vi "Make_Periodic.vi"(1 "Input Array":i64[](array[numeric])=[1, 0], 4 "Periods":u64=1) -> (15 "Output Array":i64[](array[numeric])=[1, 0], 18 "Output Length":u64=2)   [LabVIEW 2014]
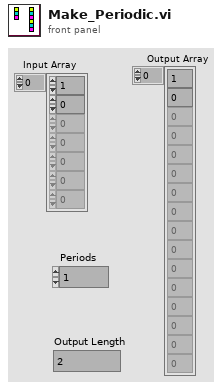
[diagram p1: front panel]
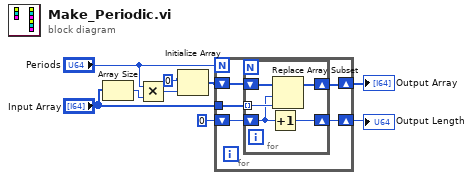
[diagram p0: block diagram]
diagram:
  n1 = Array Size(array="Input Array") -> (size(s)=w6:i32)
  n2 = Multiply(x="Periods", y=w6) -> (x*y=w4:u64)
  n3 = Initialize Array(i64 0 ("element"), w4) -> (w8:i64[])
  n4 = for {
    N: "Periods" -> [_]
    shift-right: [w12] -> w3
    shift-left: w8 -> [w13]
    tunnel: "Input Array" -> [w14]
    shift-right: [w10] -> w1
    shift-left: u64 0 ("element") -> [w11]
    n5 = for {
      tunnel: w14 -> [w17] mode=indexing
      shift-right: [w18] -> w12
      shift-left: w13 -> [w19]
      shift-right: [w16] -> w10
      shift-left: w11 -> [w15]
      n6 = Increment(x=w15) -> (x+1=w16:u64)
      n7 = Replace Array Subset(array=w19, new element=w17, index=w15) -> (w18:i64[])
    }
  }
  "Output Array" <- w3
  "Output Length" <- w1
